vi "First Step.vi"(8 "error in (no error)":errorcluster, 11 "Translation Stage Fine.lvclass in":refnum<class "Translation Stage Fine.lvclass">) -> (0 "error out":errorcluster, 2 "Current Position":dbl, 3 "Translation Stage Fine.lvclass out":refnum<class "Translation Stage Fine.lvclass">)   [LabVIEW 2017, in "Translation Stage Fine.lvclass"]
doc: "(Dynamic) Reset the instrument and prepare to scan. Go to step #0 - the first step. If desired, the scanner may do this in a different way than usual (i.e. by preparing to move a long distance, or reset to home position.)"
uses:
  Translation Stage Fine.lvclass
  Global/GPIB Numbers.vi
  Scanner/Scanner.lvclass
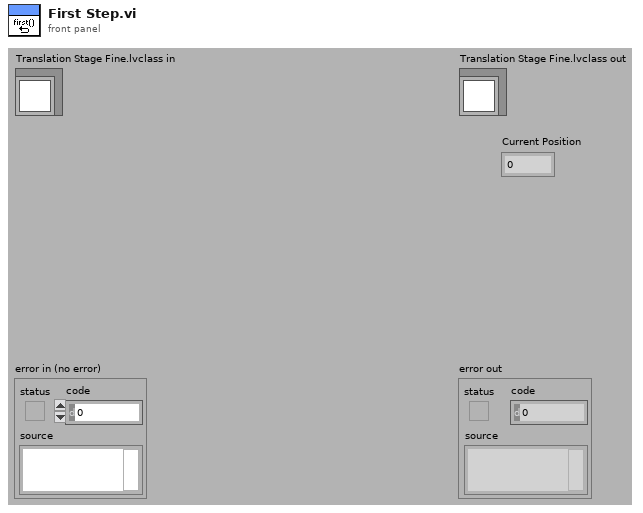
[diagram p1: front panel]
types:
  T1 = typedef "GPIB Type Def.ctl" = cluster{"Name":string, "bus":dbl, "GPIB":dbl, "GPIB as string":string, "byte":i32, "VISA Resource Name":refnum<visa-resource-name>}
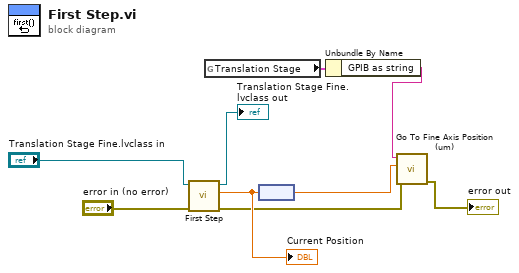
[diagram p0: block diagram]
diagram:
  n1 = call-parent "First Step.vi"("error in (no error)"="error in (no error)", "Scanner.lvclass in"="Translation Stage Fine.lvclass in") -> ("error out"=w2:errorcluster, "Current Position"=w6:dbl, "Scanner.lvclass out"=→"Translation Stage Fine.lvclass out":refnum<class "Translation Stage Fine.lvclass">)  [unwired: 7 in]
  "Current Position" <- w6
  n2 = global read "GPIB Numbers.vi" "Translation Stage"() -> (w5:T1)
  n3 = node(w6) -> (w3:dbl[unit])
  n4 = Unbundle By Name(w5) -> ("GPIB as string"=w4:string)
  n5 = call "Go To Fine Axis Position (um).vi"("error in"=w2, "Fine Axis Position (um)"=w3, "GPIB # (in): def. 6"=w4) -> ("error out"=→"error out":errorcluster)  [unwired: 7 in, 1 out]
